vi "PROIECT.vi"(3 "stop 2":bool, 11 "Boolean 2":bool) -> ()   [LabVIEW 2015]
uses:
  <vilib>/userdefined/High Color/IMAQdx.ctl
  <vilib>/vision/driver/NI_Vision_Acquisition_Software.lvlib
panel:
  out "Image":T1(plugin-control)
  in  "Boolean":bool
  in  "stop":bool
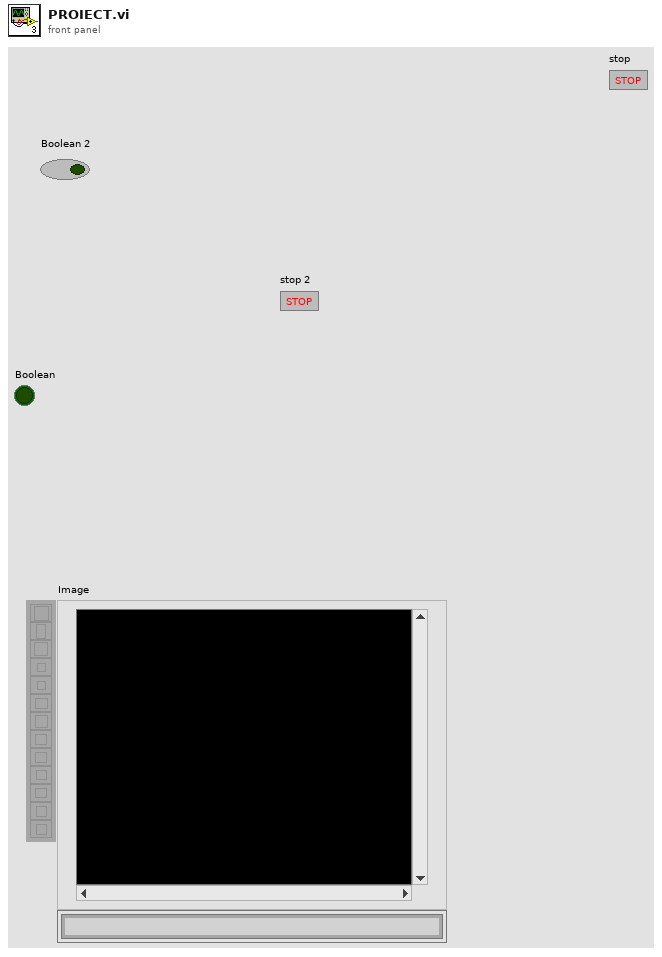
[diagram p1: front panel]
types:
  T1 = typedef "IMAQ Image.ctl" = refnum<image>
  T2 = typedef "IMAQdx.ctl" = refnum<k21>
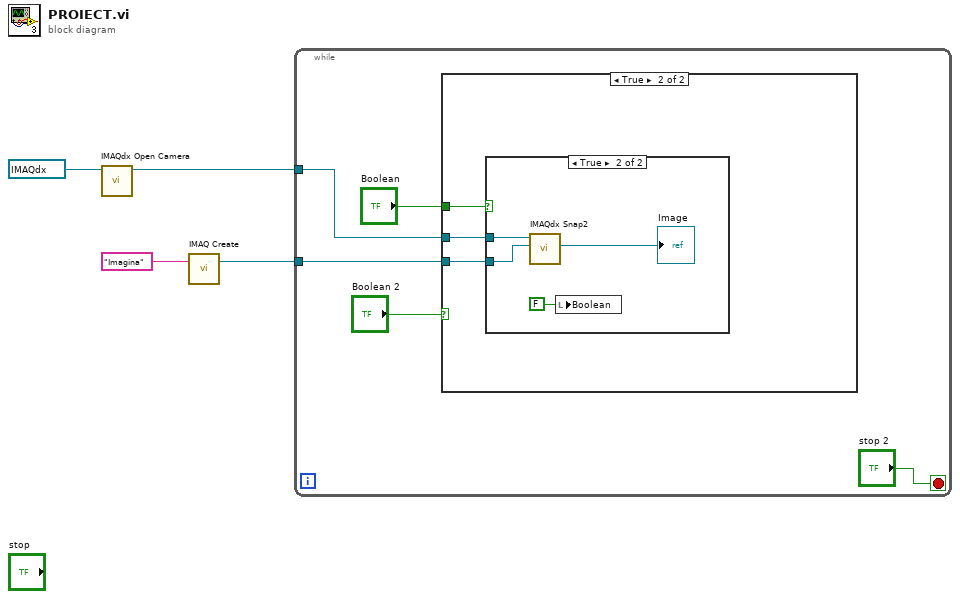
[diagram p0: block diagram]
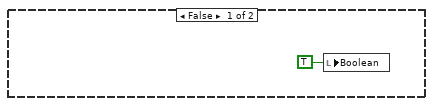
[diagram p2: hidden frame]
diagram:
  n1 = call <vilib>:"IMAQdx Open Camera.vi"("Session In"=T2 "cam0") -> ("Session Out"=w2:T2)  [unwired: 9 in, 1 out]
  n2 = call "IMAQ Create"("Image Name"="Imagina") -> ("New Image"=w1:T1)  [unwired: 4 in, 1 out]
  n3 = while {
    tunnel: w2 -> [w6]
    tunnel: w1 -> [w5]
    stop <- "stop 2" stop-if-true
    n4 = case shown="True" "Boolean 2" {
      tunnel: "Boolean" -> [_ w13]
      tunnel: w6 -> [_ w12]
      tunnel: w5 -> [_ w11]
      frame False {
        n5 = local write "Boolean"(TRUE) -> ()
      }
      frame True {
        n6 = case shown="True" w13 {
          tunnel: w12 -> [_ w16]
          tunnel: w11 -> [_ w15]
          frame False {
          }
          frame True {
            n7 = call <vilib>:"IMAQdx Snap2.vi"("Image In"=w15, "Session In"=w16) -> ("Image Out"=→"Image":T1)  [unwired: 7 in, 2 out]
            n8 = local write "Boolean"(FALSE) -> ()
          }
        }
      }
    }
  }
